vi "Multi Instrument Do Core.vi"(8 "error in (no error)":errorcluster, 10 "Actor in":refnum<class "Actor.lvclass">, 11 "Instrument Msg in":refnum<class "Multi Instrument Msg.lvclass">) -> (0 "error out":errorcluster, 1 "Data":refnum<class "Data.lvclass">, 2 "Actor out":refnum<class "Actor.lvclass">, 3 "Instrument Msg out":refnum<class "Multi Instrument Msg.lvclass">)   [LabVIEW 2020, in "Instrument Handler.lvlib" / "Multi Instrument Msg.lvclass"]
doc: "Message interaction with multiple instruments is handled by the Multi Instrument Do Core.\n\nMulti Instrument Msgs contains the Cores of all the Owners they require. Keep this in mind if the message wire is branched. Incorrect synchronization of nested Multi Instrument Msgs can lead to deadlocks if wire branching is used incorrectly!\n\nThe default implementation does nothing."
uses:
  Multi Instrument Msg/Multi Instrument Msg.lvclass
  PPL/HDH.Actor Framework.Core.Actor.lvlibp/1abvi3w/vi.lib/ActorFramework/Actor/Actor.lvclass
  PPL/HDH.Data.Generic.lvlibp/Data.lvclass
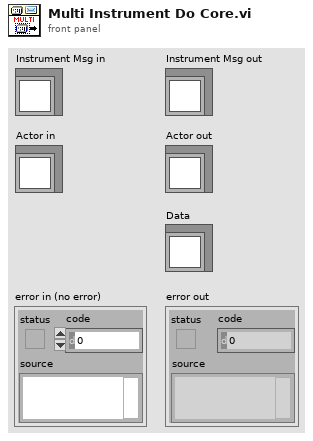
[diagram p1: front panel]
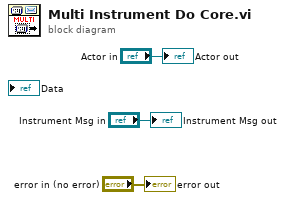
[diagram p0: block diagram]
diagram:
  "error out" <- "error in (no error)"
  "Instrument Msg out" <- "Instrument Msg in"
  "Actor out" <- "Actor in"
